vi "Actor Core.vi"(8 "error in":errorcluster, 11 "My Application":refnum<class "Main.lvclass">) -> (0 "error out":errorcluster, 3 "Actor out":refnum<class "Actor.lvclass">)   [LabVIEW 2018, in "Main.lvlib" / "Main.lvclass"]
doc: "This is Actor Core.vi, the main message handling loop for Actors. An actor usually just sits in this loop and processes messages as they arrive. Any error returned by the message Do.vi call will stop the loop, with error code 43 as the canonical signal to stop with no error sent to caller. Descendants may override that in Handle Error.vi."
uses:
  Main.lvclass
  C:/Program Files/National Instruments/LabVIEW 2018/vi.lib/MGI/Panel Manager/Panel Actor/Panel Actor/Panel Actor.lvclass
  <vilib>/ActorFramework/Actor/Actor.lvclass
  Main.lvclass/Main.ctl
  <vilib>/ActorFramework/Message Enqueuer/Message Enqueuer.lvclass/Message Enqueuer.ctl
  Main Messages/Launch Actors Msg/Launch Actors Msg.lvclass/Launch Actors Msg.ctl
  <vilib>/ActorFramework/Message Enqueuer/Enqueue.vi
  <vilib>/ActorFramework/Stop Msg/Stop Msg.lvclass
  C:/Program Files/National Instruments/LabVIEW 2018/vi.lib/ActorFramework/Message/Message.lvclass
  Main Messages/Launch Actors Msg/Launch Actors Msg.lvclass
  <vilib>/ActorFramework/Message Priority Queue/Priority Enqueue.vi
  <vilib>/MGI/Panel Manager/Panel Actor/Panel Actor/Panel Actor.lvclass
  Main.lvlib
  Main Messages/Set Print Speeds Msg/Set Print Speeds Msg.lvclass
  Main Messages/Quit Actors Msg/Quit Actors Msg.lvclass
panel:
  in  "Tab Control":enum32{"Operation", "Settings", "Debug"}(tab)
  in  "Feeder Selector":u16(ring) items=["Primary Feeder", "Secondary Feeder"]
  in  "Print Values":T1={"Screw"=1, "Inner"=0.0, "Outer"=0.0, "Mixer"=0.0} {"Mixer" scale=0.075..0.095; "Screw" items=["0%"=1, "25%"=225, "50%"=450, "75%"=675, "100%"=900]}
  in  "Quit Actors":T2
  in  "Restart Actors":T2
  in  "Physical Channels":T3={"DAQ"="Dev3", "Primary Mixer"="Dev3/ctr0", "Primary Screw"="Dev3/ctr1", "Primary Solenoid"="Dev3/port0/line0", "Inner Flow"="COM2", "Outer Flow"="COM1", "Chamber Pressure"="Dev3/ai1", "Feeder Pressure"="Dev3/ai2", "Stage"="COM4"}
  in  "Stop":bool
  # "Pressure Readings"
  # "Mass Flow Controllers"
  # "Stage Controls"
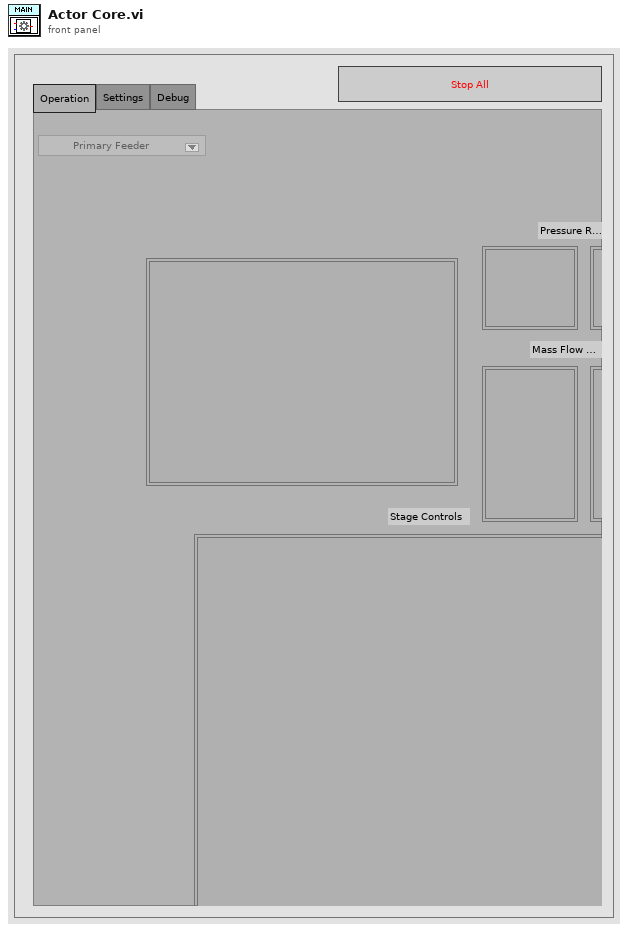
[diagram p1: front panel]
types:
  T1 = cluster{"Screw":u16, "Inner":dbl, "Outer":dbl, "Mixer":dbl}
  T2 = cluster{"Feeder":bool, "Chamber Pressure":bool, "Feeder Pressure":bool, "Inner Flow":bool, "Outer Flow":bool, "Stage":bool}
  T3 = cluster{"DAQ":tag, "Primary Mixer":tag, "Primary Screw":tag, "Primary Solenoid":tag, "Inner Flow":refnum<visa-resource-name>, "Outer Flow":refnum<visa-resource-name>, "Chamber Pressure":tag, "Feeder Pressure":tag, "Stage":refnum<visa-resource-name>}
  T4 = enum16{"Outer MFC", "Inner MFC", "Chamber Pressure", "Feeder Pressure", "Stage", "Primary Feeder", "Secondary Feeder", "All"}
  T5 = enum8{"Enabled", "Disabled", "Disabled and Grayed Out"}
  T6 = cluster{"Event Registration Refnum":refnum<event-registration>, "Pnl Actor":refnum<event-registration>}
  T7 = enum16{"Mixer", "Screw", "Inner MFC", "Outer MFC"}
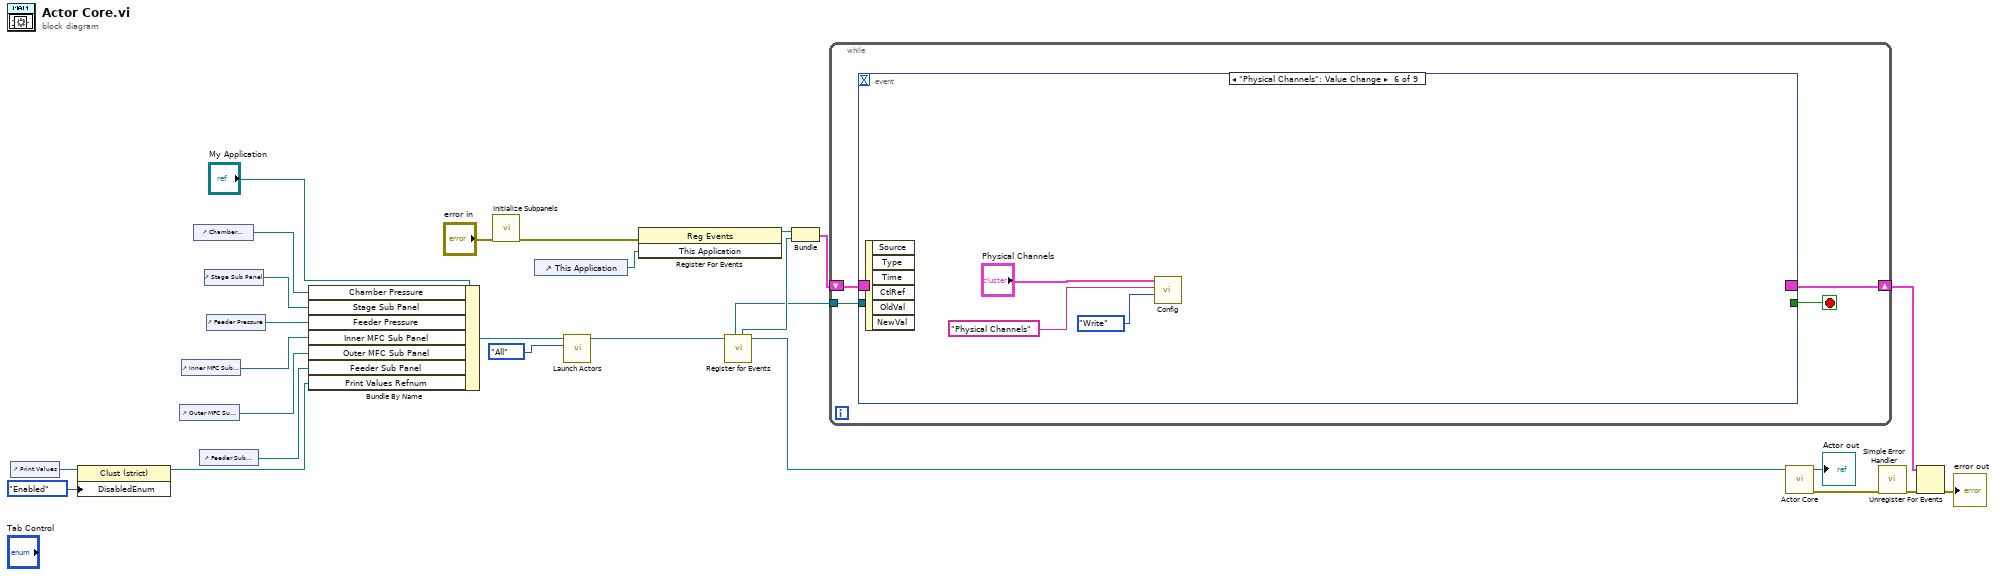
[diagram p0: block diagram]
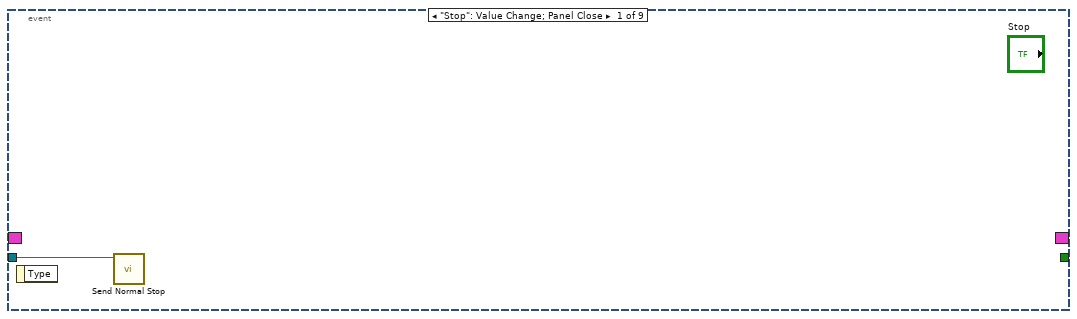
[diagram p2: hidden frame]
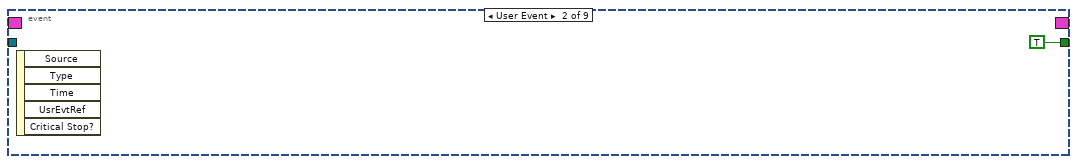
[diagram p3: hidden frame]
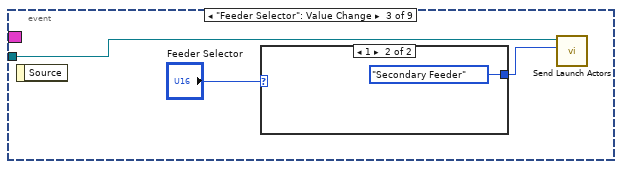
[diagram p4: hidden frame]
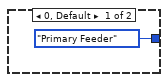
[diagram p5: hidden frame]
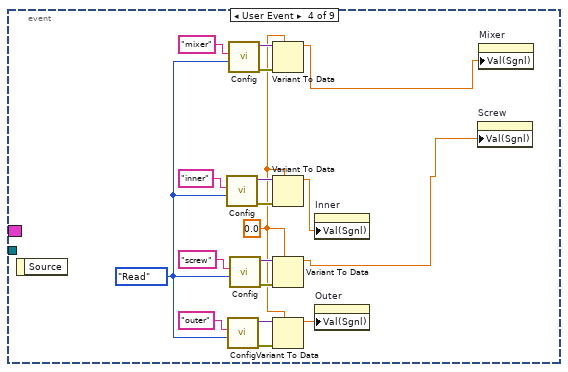
[diagram p6: hidden frame]
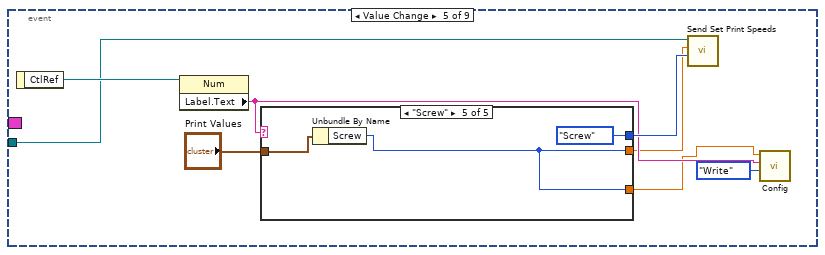
[diagram p7: hidden frame]
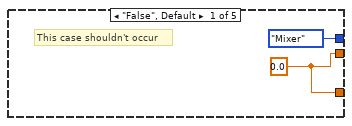
[diagram p8: hidden frame]
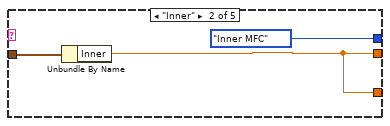
[diagram p9: hidden frame]
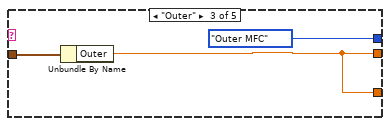
[diagram p10: hidden frame]
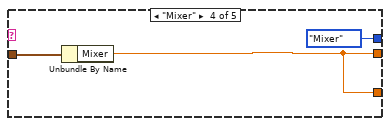
[diagram p11: hidden frame]
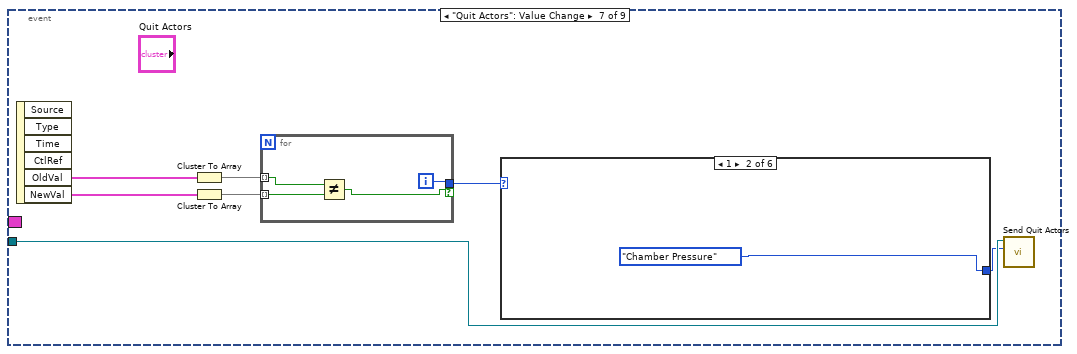
[diagram p12: hidden frame]
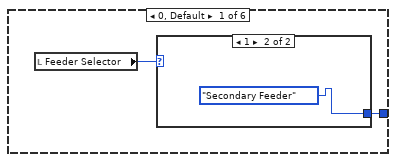
[diagram p13: hidden frame]
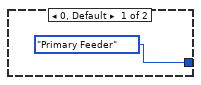
[diagram p14: hidden frame]
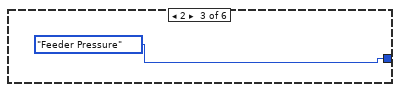
[diagram p15: hidden frame]
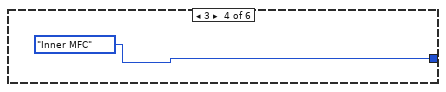
[diagram p16: hidden frame]
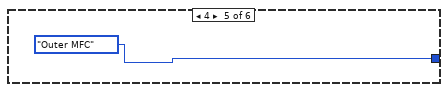
[diagram p17: hidden frame]
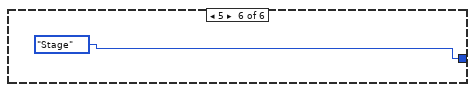
[diagram p18: hidden frame]
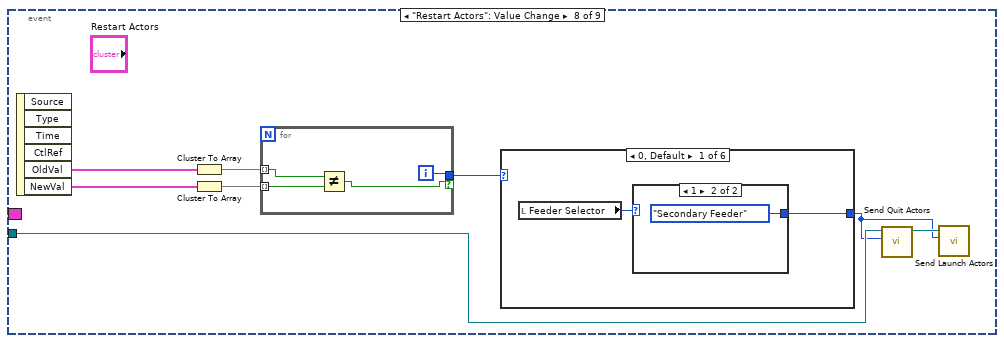
[diagram p19: hidden frame]
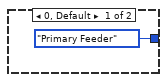
[diagram p20: hidden frame]
diagram:
  n1 = control-ref of="Print Values"() -> (w15:refnum<vi>)
  n2 = property class="Clust (strict)"(reference=w15, "DisabledEnum"=T5."Enabled" ("Disabled")) -> (reference out=w6:refnum<vi>)  [unwired: 1 in, 1 out]
  n3 = control-ref of="Outer MFC Sub Panel"() -> (w7:refnum<vi>)
  n4 = control-ref of="Inner MFC Sub Panel"() -> (w8:refnum<vi>)
  n5 = control-ref of="Chamber Pressure"() -> (w9:refnum<vi>)
  n6 = control-ref of="Feeder Sub Panel"() -> (w12:refnum<vi>)
  n7 = control-ref of="Stage Sub Panel"() -> (w11:refnum<vi>)
  n8 = control-ref of="Feeder Pressure"() -> (w10:refnum<vi>)
  n9 = Bundle By Name(cluster="My Application", "Chamber Pressure"=w9, "Stage Sub Panel"=w11, "Feeder Pressure"=w10, "Inner MFC Sub Panel"=w8, "Outer MFC Sub Panel"=w7, "Feeder Sub Panel"=w12, "Print Values Refnum"=w6) -> (w2:refnum<class "Main.lvclass">)
  n10 = call "Initialize Subpanels.vi"("error in (no error)"="error in") -> ("error out"=w1:errorcluster)  [unwired: 10 in]
  n11 = control-ref of="This Application"() -> (w21:refnum<vi>)
  n12 = call "Launch Actors.vi"("Actor"=T4."All", "Main.lvlib:Main.lvclass"=w2) -> ("Main.lvlib:Main.lvclass 2"=w5:refnum<class "Main.lvclass">)  [unwired: 8 in, 1 out]
  n13 = register-events(error in=w1, w21) -> (reference out=w18:refnum<event-registration>)  [unwired: 1 in, 1 out]
  n14 = call <vilib>:"Register for Events.vi"("Panel Actor in"=w5) -> ("Panel Actor out"=w4:refnum<class "Main.lvclass">, "Pnl Actor"=w17:refnum<event-registration>, "Self Enqueuer"=w16:refnum<class "Message Enqueuer.lvclass">)  [unwired: 7 in, 1 out]
  n15 = Bundle("Event Registration Refnum"=w18, "Pnl Actor"=w17) -> (w19:T6)  [unwired: 1 in]
  n16 = while {
    shift-right: [w28] -> w24
    shift-left: w19 -> [w29]
    tunnel: w16 -> [w27]
    stop <- w30 stop-if-true
    n17 = event shown="[5] \"Physical Channels\": Value Change" {
      selector: w29 -> [_ _ _ _ _ _ _ _ _]
      dyn-events: [_ _ _ _ _ _ _ _ _] -> w28
      timeout: _ -> [_ _ _ _ _ _ _ _ _]
      tunnel: [_ TRUE ("stop signal") _ _ _ _ _ _ _] -> w30
      tunnel: w27 -> [w31 _ w34 _ w61 _ w82 w103 _]
      event "Stop": Value Change; Panel Close {
        n18 = event-data() -> ()  [unwired: 1 in, 1 out]
        n19 = call <vilib>:"Send Normal Stop.vi"("Message Enqueuer"=w31) -> ()  [unwired: 10 in, 1 out]
      }
      event User Event {
        n20 = event-data() -> ()  [unwired: 1 in, 5 out]
      }
      event "Feeder Selector": Value Change {
        n21 = event-data() -> ()  [unwired: 1 in, 1 out]
        n22 = case shown="1" "Feeder Selector" {
          tunnel: [T4."Primary Feeder" ("Actor") T4."Secondary Feeder" ("Actor")] -> w33
          frame 0, Default {
          }
          frame 1 {
          }
        }
        n23 = call "Send Launch Actors.vi"("Actor"=w33, "Message Enqueuer in"=w34) -> ()  [unwired: 8 in, 2 out]
      }
      event User Event {
        w41 = 0.0
        w51 = enum16{"Read", "Write"}."Read" ("Action")
        n24 = event-data() -> ()  [unwired: 1 in, 1 out]
        n25 = call "Config.vi"("Action"=w51, "Variable Name"="inner") -> ("error out"=w50:errorcluster, "Variable Value Out"=w49:variant)  [unwired: 8 in]
        n26 = call "Config.vi"("Action"=w51, "Variable Name"="outer") -> ("error out"=w45:errorcluster, "Variable Value Out"=w46:variant)  [unwired: 8 in]
        n27 = call "Config.vi"("Action"=w51, "Variable Name"="mixer") -> ("error out"=w48:errorcluster, "Variable Value Out"=w47:variant)  [unwired: 8 in]
        n28 = call "Config.vi"("Action"=w51, "Variable Name"="screw") -> ("error out"=w43:errorcluster, "Variable Value Out"=w44:variant)  [unwired: 8 in]
        n29 = Variant To Data(error in=w48, type=w41, Variant=w47) -> (data=w39:dbl)  [unwired: 1 out]
        n30 = Variant To Data(error in=w50, type=w41, Variant=w49) -> (data=w40:dbl)  [unwired: 1 out]
        n31 = Variant To Data(error in=w43, type=w41, Variant=w44) -> (data=w38:dbl)  [unwired: 1 out]
        n32 = Variant To Data(error in=w45, type=w41, Variant=w46) -> (data=w42:dbl)  [unwired: 1 out]
        n33 = property on="Inner" class="DigNum (strict)"("Val(Sgnl)"=w40) -> ()  [unwired: 2 in, 2 out]
        n34 = property on="Outer" class="DigNum (strict)"("Val(Sgnl)"=w42) -> ()  [unwired: 2 in, 2 out]
        n35 = property on="Screw" class="Ring (strict)"("Val(Sgnl)"=w38) -> ()  [unwired: 2 in, 2 out]
        n36 = property on="Mixer" class="Knob (strict)"("Val(Sgnl)"=w39) -> ()  [unwired: 2 in, 2 out]
      }
      event "Print Values.Mixer", "Print Values.Outer", "Print Values.Screw", "Print Values.Inner": Value Change {
        n37 = event-data() -> ("CtlRef"=w63:refnum<vi>)  [unwired: 1 in]
        n38 = property class="Num"(reference=w63) -> ("Label.Text"=w59:string)  [unwired: 1 in, 2 out]
        n39 = case shown="\"Screw\"" w59 {
          tunnel: "Print Values" -> [_ w68 w71 w74 w77]
          tunnel: [w64 w66 w69 w72 w75] -> w56
          tunnel: [T7."Mixer" ("Actor") T7."Inner MFC" ("Actor") T7."Outer MFC" ("Actor") T7."Mixer" ("Actor") T7."Screw" ("Actor")] -> w60
          tunnel: [w64 w66 w69 w72 w75] -> w57
          frame "False", Default {
            w64 = 0.0 ("Outer")
            # "This case shouldn't occur"
          }
          frame "Inner" {
            n40 = Unbundle By Name(w68) -> ("Inner"=w66:dbl)
          }
          frame "Outer" {
            n41 = Unbundle By Name(w71) -> ("Outer"=w69:dbl)
          }
          frame "Mixer" {
            n42 = Unbundle By Name(w74) -> ("Mixer"=w72:dbl)
          }
          frame "Screw" {
            n43 = Unbundle By Name(w77) -> ("Screw"=w75:u16)
          }
        }
        n44 = call "Send Set Print Speeds.vi"("Actor"=w60, "Speed"=w56, "Message Enqueuer in"=w61) -> ()  [unwired: 7 in, 2 out]
        n45 = call "Config.vi"("Action"=enum16{"Read", "Write"}."Write", "Variable Name"=w59, "Variable Value In"=w57) -> ()  [unwired: 7 in, 2 out]
      }
      event "Physical Channels": Value Change {
        n46 = event-data() -> ()  [unwired: 1 in, 6 out]
        n47 = call "Config.vi"("Action"=enum16{"Read", "Write"}."Write", "Variable Name"="Physical Channels", "Variable Value In"="Physical Channels") -> ()  [unwired: 7 in, 2 out]
      }
      event "Quit Actors": Value Change {
        n48 = event-data() -> ("OldVal"=w87:T2, "NewVal"=w86:T2)  [unwired: 1 in, 4 out]
        n49 = Cluster To Array(cluster=w87) -> (array=w85:bool[])
        n50 = Cluster To Array(cluster=w86) -> (array=w84:bool[])
        n51 = for {
          tunnel: w85 -> [w100] mode=indexing
          tunnel: w84 -> [w99] mode=indexing
          tunnel: [w98] -> w83 if=w97
          i -> [w98]
          n52 = Not Equal?(x=w100, y=w99) -> (x != y?=w97:bool)
        }
        n53 = case shown="1" w83 {
          tunnel: [w88 T4."Chamber Pressure" ("Actor") T4."Feeder Pressure" ("Actor") T4."Inner MFC" ("Actor") T4."Outer MFC" ("Actor") T4."Stage" ("Actor")] -> w81
          frame 0, Default {
            n54 = local read "Feeder Selector"() -> (w89:u16)
            n55 = case shown="1" w89 {
              tunnel: [T4."Primary Feeder" ("Actor") T4."Secondary Feeder" ("Actor")] -> w88
              frame 0, Default {
              }
              frame 1 {
              }
            }
          }
          frame 1 {
          }
          frame 2 {
          }
          frame 3 {
          }
          frame 4 {
          }
          frame 5 {
          }
        }
        n56 = call "Send Quit Actors.vi"("Actor"=w81, "Message Enqueuer in"=w82) -> ()  [unwired: 8 in, 2 out]
      }
      event "Restart Actors": Value Change {
        n57 = event-data() -> ("OldVal"=w108:T2, "NewVal"=w107:T2)  [unwired: 1 in, 4 out]
        n58 = Cluster To Array(cluster=w108) -> (array=w106:bool[])
        n59 = Cluster To Array(cluster=w107) -> (array=w105:bool[])
        n60 = for {
          tunnel: w106 -> [w121] mode=indexing
          tunnel: w105 -> [w120] mode=indexing
          tunnel: [w119] -> w104 if=w118
          i -> [w119]
          n61 = Not Equal?(x=w121, y=w120) -> (x != y?=w118:bool)
        }
        n62 = case shown="0, Default" w104 {
          tunnel: [w109 T4."Chamber Pressure" ("Actor") T4."Feeder Pressure" ("Actor") T4."Inner MFC" ("Actor") T4."Outer MFC" ("Actor") T4."Stage" ("Actor")] -> w101
          frame 0, Default {
            n63 = local read "Feeder Selector"() -> (w110:u16)
            n64 = case shown="1" w110 {
              tunnel: [T4."Primary Feeder" ("Actor") T4."Secondary Feeder" ("Actor")] -> w109
              frame 0, Default {
              }
              frame 1 {
              }
            }
          }
          frame 1 {
          }
          frame 2 {
          }
          frame 3 {
          }
          frame 4 {
          }
          frame 5 {
          }
        }
        n65 = call "Send Quit Actors.vi"("Actor"=w101, "Message Enqueuer in"=w103) -> ("Message Enqueuer out"=w102:refnum<class "Message Enqueuer.lvclass">)  [unwired: 8 in, 1 out]
        n66 = call "Send Launch Actors.vi"("Actor"=w101, "Message Enqueuer in"=w102) -> ()  [unwired: 8 in, 2 out]
      }
      event Application Instance Close {
        n67 = event-data() -> ()  [unwired: 1 in, 1 out]
        n68 = call <vilib>:"DAQmx Reset Device.vi"("device in"=tag "Dev1") -> ()  [unwired: 14 in, 1 out]
      }
    }
  }
  n69 = call-parent "Actor Core.vi"("Panel Actor in"=w4) -> ("error out"=w25:errorcluster, "Actor out"=→"Actor out":refnum<class "Actor.lvclass">)  [unwired: 9 in]
  n70 = call <vilib>:"Simple Error Handler.vi"("error in (no error)"=w25) -> ("error out"=w23:errorcluster)  [unwired: 4 in, 4 out]
  n71 = Unregister For Events(event registration refnum=w24, error in=w23) -> (error out=→"error out":errorcluster)
